vi "Flatten to String.vi"(8 "error in (no error)":errorcluster, 11 "GenericSerializable in":refnum<class "GenericSerializable.lvclass">) -> (0 "error out":errorcluster, 3 "Flattened Class":string)   [LabVIEW 2020, in "Logger Examples.lvlib" / "GenericSerializable.lvclass"]
uses:
  <vilib>/gpm_packages/@cs/event-logger/Examples/GenericSerializable/GenericSerializable.lvclass
  <vilib>/gpm_packages/@cs/event-logger/Examples/GenericSerializable/GenericSerializable.lvclass/GenericSerializable.ctl
  <vilib>/Utility/Data Type/NI_Data Type.lvlib
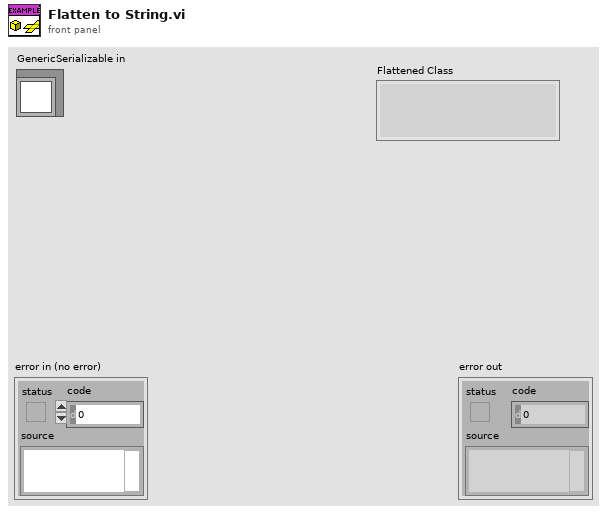
[diagram p1: front panel]
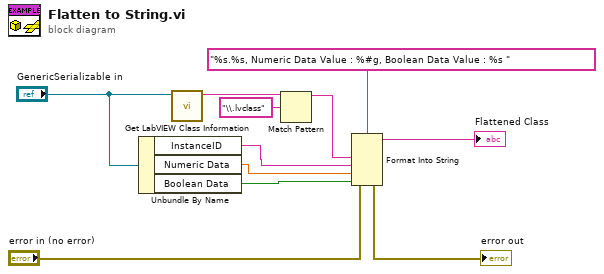
[diagram p0: block diagram]
diagram:
  n1 = Unbundle By Name("GenericSerializable in") -> ("InstanceID"=w5:string, "Numeric Data"=w6:dbl, "Boolean Data"=w8:bool)
  n2 = call <vilib>:"Get LabVIEW Class Information.vi"("variant"="GenericSerializable in") -> ("LabVIEW class file name"=w11:string)  [unwired: 8 in, 2 out]
  n3 = Match Pattern(string=w11, regular expression="\\.lvclass") -> (before substring=w4:string)  [unwired: 1 in, 3 out]
  n4 = Format Into String(format string="%s.%s, Numeric Data Value : %#g, Boolean Data Value : %s ", error in="error in (no error)", w4, w5, w6, w8) -> (resulting string=→"Flattened Class":string, error out=→"error out":errorcluster)  [unwired: 1 in]
